vi "Event Log Reference.vi"() -> ()   [LabVIEW 2022 SP3]
uses:
  <vilib>/NI/Event Logger Library/EventLog/EventLog.lvclass
panel:
  in  "Event Log Reference":refnum<class "EventLog.lvclass">
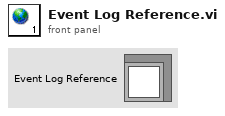
[diagram p1: front panel]
diagram:
